vi "Write status.vi"(8 "error in (no error)":errorcluster, 10 "status":bool, 11 "TCSCommand in":refnum<class "TCSCommand.lvclass">) -> (0 "error out":errorcluster, 3 "TCSCommand out":refnum<class "TCSCommand.lvclass">)   [LabVIEW 2014, in "TCSDataDefinitions.lvlib" / "TCSCommand.lvlib" / "TCSCommand.lvclass"]
uses:
  TCSCommand.lvclass
  TCSCommand.lvclass/TCSCommand.ctl
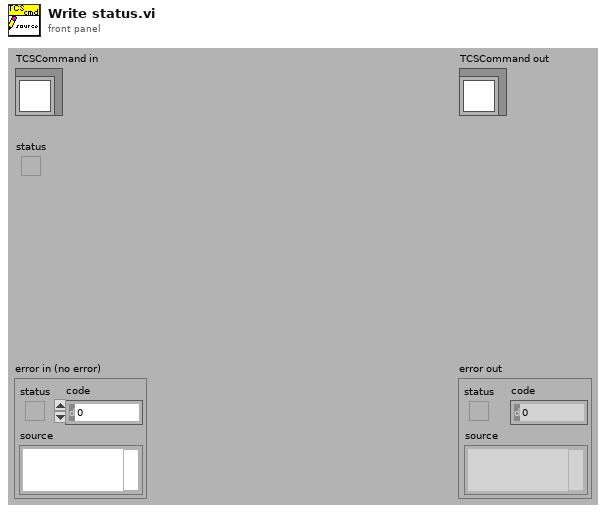
[diagram p1: front panel]
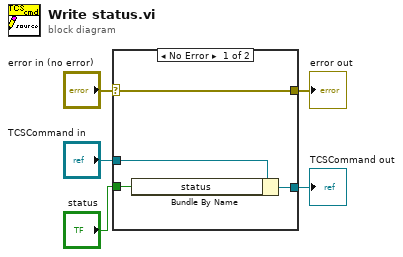
[diagram p0: block diagram]
diagram:
  n1 = case shown="No Error" "error in (no error)" {
    selector: "error in (no error)" -> [w9 w10]
    tunnel: [w9 w10] -> w4
    tunnel: [w7 w11] -> w2
    tunnel: "TCSCommand in" -> [w8 w11]
    tunnel: "status" -> [w6 _]
    frame No Error {
      n2 = Bundle By Name(cluster=w8, "status"=w6) -> (w7:refnum<class "TCSCommand.lvclass">)
    }
    frame Error {
    }
  }
  "error out" <- w4
  "TCSCommand out" <- w2
